vi "Insert DB data.vi"(6 "index":i32, 7 "Data":string[](array[string]), 8 "error in (no error)":errorcluster caption="错误输入（无错误）", 10 "table":string, 11 "Connncet State":T1) -> (0 "error out":errorcluster caption="错误输出", 2 "state":bool, 3 "Connect State":T1)   [LabVIEW 2014]
uses:
  Ctr/Constr.ctl
  <vilib>/addons/database/Connection.llb/Conn ObjectReference.ctl
  <vilib>/addons/database/NI_Database_API.lvlib
  Ctr/Conneect State.ctl
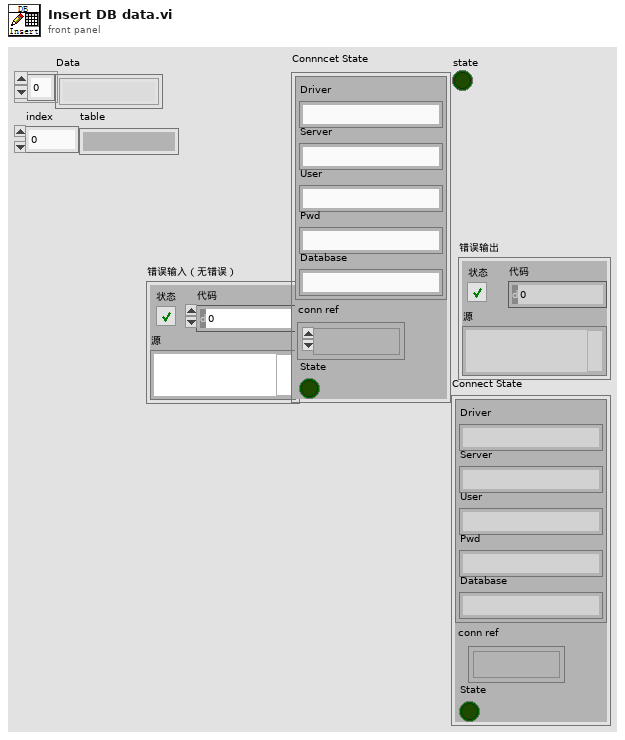
[diagram p1: front panel]
types:
  T1 = typedef "Conneect State.ctl" = cluster{"Constr":T2, "conn ref":T3, "State":bool}
  T2 = typedef "Constr.ctl" = cluster{"Driver":string, "Server":string, "User":string, "Pwd":string, "Database":string}
  T3 = typedef "NI_Database_API.lvlib/Conn ObjectReference.ctl" = refnum<k1>
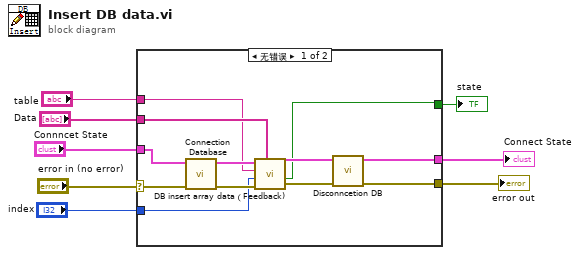
[diagram p0: block diagram]
diagram:
  n1 = case shown="无错误" "error in (no error)" {
    selector: "error in (no error)" -> [w20 w21]
    tunnel: "Connncet State" -> [w19 w22]
    tunnel: "Data" -> [w16 _]
    tunnel: "index" -> [w15 _]
    tunnel: "table" -> [w14 _]
    tunnel: [w11 w21] -> w3
    tunnel: [w10 w22] -> w2
    tunnel: [w9 _] -> w1
    frame No Error {
      n2 = call "Connection Database.vi"("error in (no error)"=w20, "Connncet State"=w19) -> ("error out"=w18:errorcluster, "Connncet State out"=w17:T1)  [unwired: 8 in]
      n3 = call "DB insert array data（Feedback).vi"("Data"=w16, "error in (no error)"=w18, "index"=w15, "table"=w14, "Connncet State"=w17) -> ("error out"=w13:errorcluster, "state"=w9:bool, "Connncet State out"=w12:T1)  [unwired: 4 in]
      n4 = call "Disconncetion DB.vi"("error in (no error)"=w13, "Connncet State"=w12) -> ("error out"=w11:errorcluster, "Connect State"=w10:T1)  [unwired: 8 in]
    }
    frame Error {
    }
  }
  "error out" <- w3
  "Connect State" <- w2
  "state" <- w1
